vi "Cleanup BLRL Source.vi"(8 "error in (no error)":errorcluster, 11 "User BluelinesRedlines in":refnum<class "User BluelinesRedlines.lvclass">) -> (0 "error out":errorcluster, 3 "User BluelinesRedlines out":refnum<class "User BluelinesRedlines.lvclass">)   [LabVIEW 2020, in "VolatusGUIElements.lvlib" / "User BluelinesRedlines.lvclass"]
uses:
  User BluelinesRedlines.lvclass
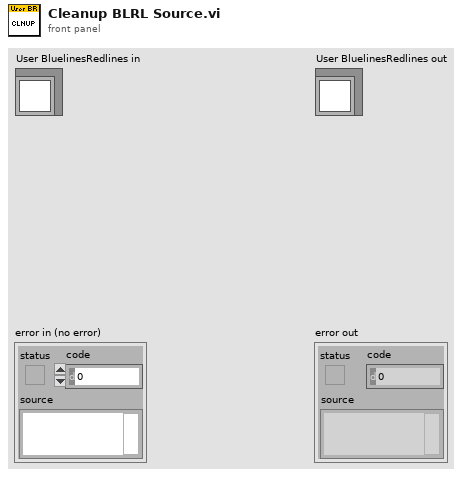
[diagram p1: front panel]
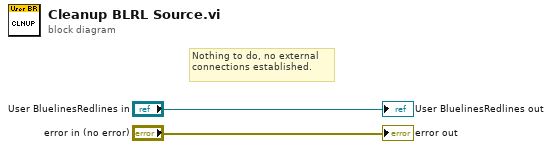
[diagram p0: block diagram]
diagram:
  # "Nothing to do, no external connections established."
  "error out" <- "error in (no error)"
  "User BluelinesRedlines out" <- "User BluelinesRedlines in"
